vi "FinBuild4.vi"   [LabVIEW 2015]
uses:
  <vilib>/NXT/Block Support/NXT_InputPort.ctl
  <vilib>/NXT/Block Support/NXT_OutputPort.ctl
  <vilib>/NXT/Dual Mode Library/Sensors/Light_On.vi
  <vilib>/NXT/Dual Mode Library/Sensors/Sonar_cm.vi
  <vilib>/NXT/NXTIO Xnodes/NXTIONodeSubVIs/NXTMoveMotors.vi
  <vilib>/NXT/Dual Mode Library/Waits/Wait_Num(msec).vi
  <vilib>/NXT/Subs/LVHSConnector.ctl
  <vilib>/NXT/NXTIO Xnodes/AddressXNode/NXTIOAddress.xnode
  <vilib>/NXT/NXTIO Xnodes/NXTIOXNode/NXTIO.xnode
  <vilib>/NXT/LegoClasses/BrickReference/BrickReference.lvclass
types:
  T1 = typedef "NXT_OutputPort.ctl" = u8
  T2 = typedef "NXT_InputPort.ctl" = u32
  T3 = typedef "LVHSConnector.ctl" = refnum<class "BrickReference.lvclass">
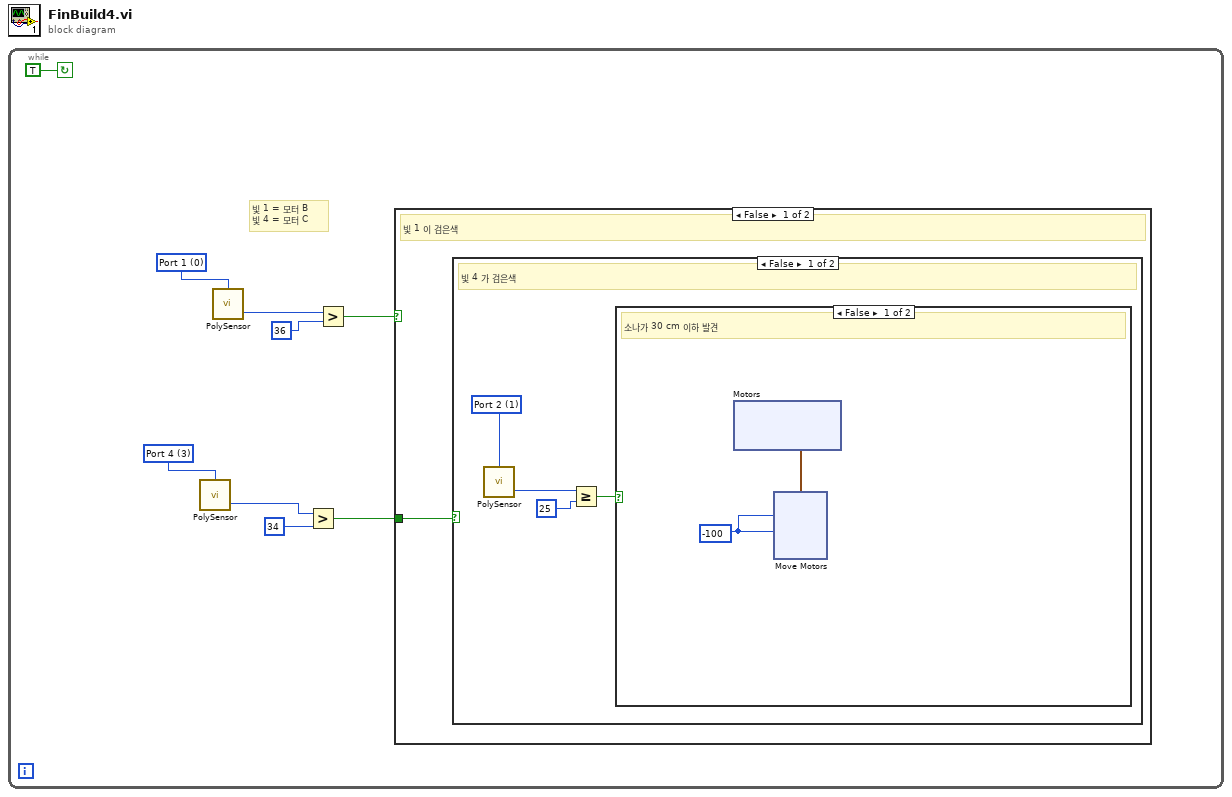
[diagram p0: block diagram]
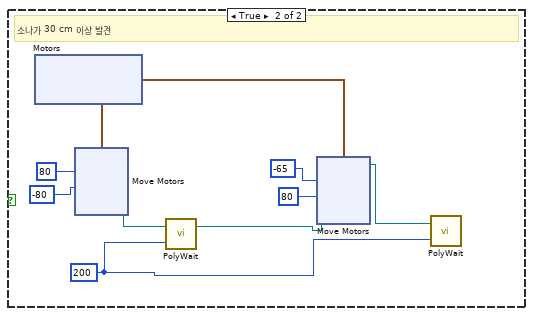
[diagram p2: hidden frame]
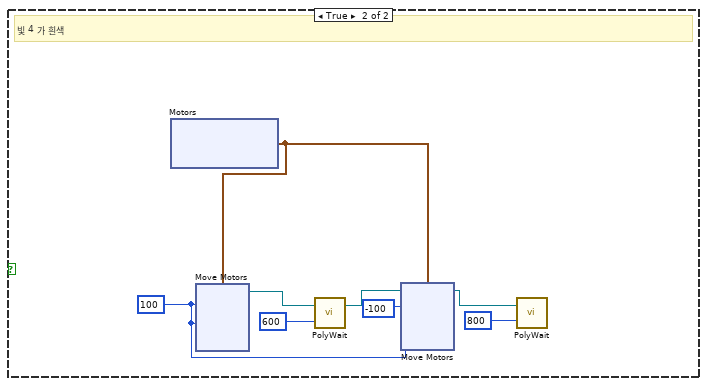
[diagram p3: hidden frame]
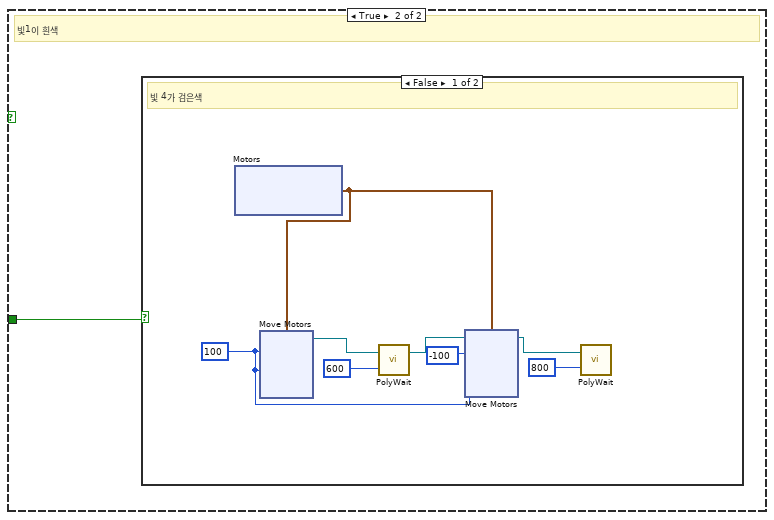
[diagram p4: hidden frame]
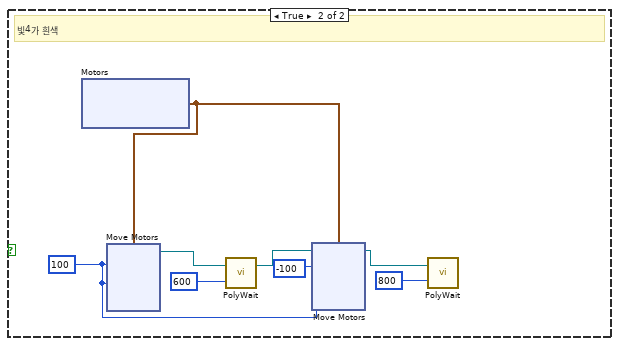
[diagram p5: hidden frame]
diagram:
  n1 = while {
    stop <- TRUE continue-if-true
    w7 = T2 0 items=["Port 1", "Port 2", "Port 3", "Port 4"] ("Port (Port 3)")
    w6 = T2 3 items=["Port 1", "Port 2", "Port 3", "Port 4"] ("Port (Port 3)")
    # "빛 1 = 모터 B\n빛 4 = 모터 C"
    n2 = call-poly <vilib>:"PolySensor.vi"("Port (Port 3)"=w6) -> ("Scaled Value"=w8:i16)  [unwired: 2 in, 1 out]
    n3 = call-poly <vilib>:"PolySensor.vi"("Port (Port 3)"=w7) -> ("Scaled Value"=w9:i16)  [unwired: 2 in, 1 out]
    n4 = Greater?(x=w8, y=i16 34) -> (0:w4:bool)
    n5 = Greater?(x=w9, y=i16 36) -> (0:w5:bool)
    n6 = case shown="False" w5 {
      tunnel: w4 -> [w10 w77]
      frame False {
        # "빛 1 이 검은색"
        n7 = case shown="False" w10 {
          frame False {
            w11 = T2 1 items=["Port 1", "Port 2", "Port 3", "Port 4"] ("Port (Port 4)")
            # "빛 4 가 검은색"
            n8 = call-poly <vilib>:"PolySensor.vi"("Port (Port 4)"=w11) -> ("Distance (cm)"=w14:i16)  [unwired: 2 in, 1 out]
            n9 = Greater Or Equal?(x=w14, y=i16 25) -> (x >= y?=w12:bool)
            n10 = case shown="False" w12 {
              frame False {
                w15 = i16 -100 ("y")
                # "소나가 30 cm 이하 발견"
                n11 = xnode "Motors"() -> ("Motor"=w16:cluster{"Port":T1, "Port":T1})
                n12 = xnode "Move Motors"("Power/Speed 2"=w15, "Power/Speed 1"=w15, "Motors"=w16) -> ()  [unwired: 1 in, 1 out]
              }
              frame True {
                w33 = i16 200 ("y")
                # "소나가 30 cm 이상 발견"
                n13 = xnode "Motors"() -> ("Motor"=w34:cluster{"Port":T1, "Port":T1})
                n14 = xnode "Move Motors"("Power/Speed 2"=i16 -80 ("y"), "Power/Speed 1"=i16 80 ("y"), "Motors"=w34) -> ("NXT/EV3"=w28:T3)  [unwired: 1 in]
                n15 = call-poly <vilib>:"PolyWait.vi"("Time (100 msec)"=w33, "NXT/EV3"=w28) -> ("NXT/EV3"=w26:T3)  [unwired: 2 in]
                n16 = xnode "Move Motors"("Power/Speed 2"=i16 80 ("y"), "Power/Speed 1"=i16 -65 ("y"), "Motors"=w34, "NXT/EV3"=w26) -> ("NXT/EV3"=w27:T3)
                n17 = call-poly <vilib>:"PolyWait.vi"("Time (100 msec)"=w33, "NXT/EV3"=w27) -> ()  [unwired: 2 in, 1 out]
              }
            }
          }
          frame True {
            w52 = i16 100 ("y")
            # "빛 4 가 흰색"
            n18 = xnode "Motors"() -> ("Motor"=w59:cluster{"Port":T1, "Port":T1})
            n19 = xnode "Move Motors"("Power/Speed 2"=w52, "Power/Speed 1"=w52, "Motors"=w59) -> ("NXT/EV3"=w58:T3)  [unwired: 1 in]
            n20 = call-poly <vilib>:"PolyWait.vi"("Time (100 msec)"=i16 600 ("y"), "NXT/EV3"=w58) -> ("NXT/EV3"=w57:T3)  [unwired: 2 in]
            n21 = xnode "Move Motors"("Power/Speed 2"=w52, "Power/Speed 1"=i16 -100 ("y"), "Motors"=w59, "NXT/EV3"=w57) -> ("NXT/EV3"=w56:T3)
            n22 = call-poly <vilib>:"PolyWait.vi"("Time (100 msec)"=i16 800 ("y"), "NXT/EV3"=w56) -> ()  [unwired: 2 in, 1 out]
          }
        }
      }
      frame True {
        # "빛1이 흰색"
        n23 = case shown="False" w77 {
          frame False {
            w78 = i16 100 ("y")
            # "빛 4가 검은색"
            n24 = xnode "Motors"() -> ("Motor"=w85:cluster{"Port":T1, "Port":T1})
            n25 = xnode "Move Motors"("Power/Speed 2"=w78, "Power/Speed 1"=w78, "Motors"=w85) -> ("NXT/EV3"=w84:T3)  [unwired: 1 in]
            n26 = call-poly <vilib>:"PolyWait.vi"("Time (100 msec)"=i16 600 ("y"), "NXT/EV3"=w84) -> ("NXT/EV3"=w83:T3)  [unwired: 2 in]
            n27 = xnode "Move Motors"("Power/Speed 2"=w78, "Power/Speed 1"=i16 -100 ("y"), "Motors"=w85, "NXT/EV3"=w83) -> ("NXT/EV3"=w82:T3)
            n28 = call-poly <vilib>:"PolyWait.vi"("Time (100 msec)"=i16 800 ("y"), "NXT/EV3"=w82) -> ()  [unwired: 2 in, 1 out]
          }
          frame True {
            w103 = i16 100 ("y")
            # "빛4가 흰색"
            n29 = xnode "Motors"() -> ("Motor"=w110:cluster{"Port":T1, "Port":T1})
            n30 = xnode "Move Motors"("Power/Speed 2"=w103, "Power/Speed 1"=w103, "Motors"=w110) -> ("NXT/EV3"=w109:T3)  [unwired: 1 in]
            n31 = call-poly <vilib>:"PolyWait.vi"("Time (100 msec)"=i16 600 ("y"), "NXT/EV3"=w109) -> ("NXT/EV3"=w108:T3)  [unwired: 2 in]
            n32 = xnode "Move Motors"("Power/Speed 2"=w103, "Power/Speed 1"=i16 -100 ("y"), "Motors"=w110, "NXT/EV3"=w108) -> ("NXT/EV3"=w107:T3)
            n33 = call-poly <vilib>:"PolyWait.vi"("Time (100 msec)"=i16 800 ("y"), "NXT/EV3"=w107) -> ()  [unwired: 2 in, 1 out]
          }
        }
      }
    }
  }
